vi "publisher tests Writer 9.vi"() -> ()   [LabVIEW 2018]
uses:
  publisher action.ctl
panel:
  out "Numeric":i32
  out "number":dbl
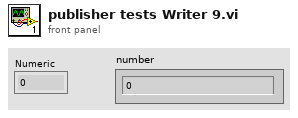
[diagram p1: front panel]
types:
  T1 = typedef "publisher action.ctl" = enum16{"set", "get", "init", "check"}
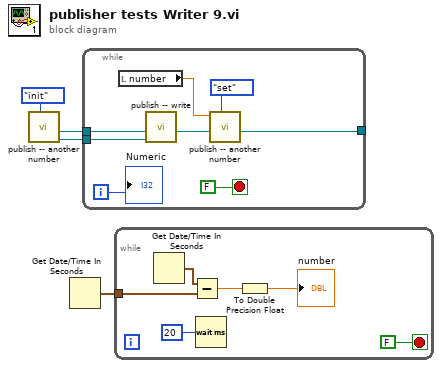
[diagram p0: block diagram]
diagram:
  n1 = call "publish -- another number.vi"("publisher action"=publisher_action."init") -> ("request event"=w2:refnum<user-event>, "recieve event"=w1:refnum<user-event>)  [unwired: 8 in, 1 out]
  n2 = Get Date/Time In Seconds() -> (seconds since 1Jan1904=w4:timestamp)
  n3 = while {
    tunnel: w2 -> [w10]
    tunnel: w1 -> [w9]
    tunnel: [w5] -> _
    i -> [w11]
    stop <- FALSE stop-if-true
    n4 = local read "number"() -> (w6:dbl)
    n5 = call "publish -- write.vi"("request event"=w10, "response event"=w9) -> ("response event OUT"=w8:refnum<user-event>)  [unwired: 9 in]
    n6 = call "publish -- another number.vi"("publisher action"=publisher_action."set", "recieve event inn"=w8, "Numeric"=w6) -> ("recieve event"=w5:refnum<user-event>)  [unwired: 6 in, 2 out]
    "Numeric" <- w11
  }
  n7 = while {
    tunnel: w4 -> [w15]
    stop <- FALSE stop-if-true
    n8 = Get Date/Time In Seconds() -> (seconds since 1Jan1904=w17:timestamp)
    n9 = Subtract(x=w17, y=w15) -> (x-y=w18:dbl)
    n10 = Wait (ms)(milliseconds to wait=u32 20) -> ()  [unwired: 1 out]
    n11 = To Double Precision Float(number=w18) -> (double precision float=→"number":dbl)
  }
